vi "TaskDeinitialize.vi"(8 "error in (no error)":errorcluster, 11 "HGF_DSCVarManager in":refnum<class "HGF_DSCVarManager.lvclass">) -> (0 "error out":errorcluster, 3 "HGF_DSCVarManager out":refnum<class "HGF_DSCVarManager.lvclass">)   [LabVIEW 2012, in "HGF_DSC.lvlib" / "HGF_DSCVarManager.lvclass"]
doc: "Called by TaskLoop to deinitialize Task.\nDeletes all variables of the Manager's process and the process itself.\n\nF.Berck@gsi.de\nGSI Darmstadt 2010"
uses:
  HGF_DSCVarManager.lvclass
  HGF_DSCVarManager.lvclass/HGF_DSCVarManager.ctl
  <vilib>/lvdsc/NI_DSC.lvlib
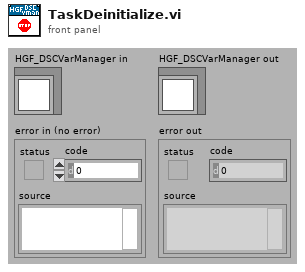
[diagram p1: front panel]
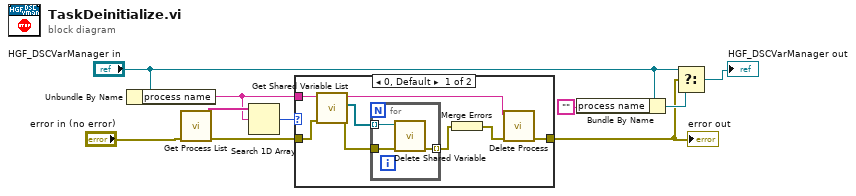
[diagram p0: block diagram]
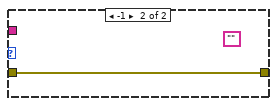
[diagram p2: hidden frame]
diagram:
  n1 = Unbundle By Name("HGF_DSCVarManager in") -> ("process name"=w2:string)
  n2 = call <vilib>:"Get Process List.vi"("error in (no error)"="error in (no error)") -> ("error out"=w7:errorcluster, "processes"=w9:string[])  [unwired: 9 in]
  n3 = Search 1D Array(1D array=w9, element=w2) -> (index of element=w8:i32)  [unwired: 1 in]
  n4 = case shown="0, Default" w8 {
    tunnel: [w11 w22] -> w3
    tunnel: w7 -> [w17 w22]
    tunnel: w2 -> [w18 _]
    frame 0, Default {
      n5 = call <vilib>:"Get Shared Variable List.vi"("error in (no error)"=w17, "process name"=w18) -> ("error out"=w14:errorcluster, "shared variables"=w15:refnum<k21>[], "process name out"=w16:string)  [unwired: 7 in]
      n6 = for {
        tunnel: w15 -> [w21] mode=indexing
        tunnel: w14 -> [w20]
        tunnel: [w19] -> w13 mode=indexing
        n7 = call <vilib>:"Delete Shared Variable.vi"("error in (no error)"=w20, "shared variable"=w21) -> ("error out"=w19:errorcluster)  [unwired: 9 in]
      }
      n8 = Merge Errors(w13) -> (w12:errorcluster)
      n9 = call <vilib>:"Delete Process.vi"("error in (no error)"=w12, "process name"=w16) -> ("error out"=w11:errorcluster)  [unwired: 9 in]
    }
    frame -1 {
      (unwired) ""
    }
  }
  "error out" <- w3
  n10 = Bundle By Name(cluster="HGF_DSCVarManager in", "process name"="") -> (w5:refnum<class "HGF_DSCVarManager.lvclass">)
  n11 = Select(t="HGF_DSCVarManager in", s=w3, f=w5) -> (s? t:f=→"HGF_DSCVarManager out":refnum<class "HGF_DSCVarManager.lvclass">)
